vi "NI-Digital Burst Pattern.vi"() -> ()   [LabVIEW 2021]
doc: "Overview\nDemonstrates bursting a pattern that uses the scan opcode and calling the History RAM Fetch Scan Cycle Numbers API."
uses:
  <instrlib>/niDigital/niDigital.llb/niDigital Selected Function.ctl
  <vilib>/Utility/file.llb/Write Delimited Spreadsheet (string).vi
  <instrlib>/niDigital/niDigital.llb/niDigital Fetch History RAM Cycle Information (1D Pin States).vi
  <instrlib>/niDigital/niDigital.llb/niDigital Configure First Failure History RAM Trigger.vi
  <instrlib>/niDigital/niDigital.llb/niDigital Load Specifications Levels and Timing (Single).vi
  <instrlib>/niDigital/niDigital.llb/niDigital Get Pattern Pin List.vi
  <instrlib>/niDigital/niDigital.llb/niDigital Get Pattern Pin Names.vi
  <instrlib>/niDigital/niDigital.llb/niDigital Burst Pattern (Pass Fail).vi
  <instrlib>/niDigital/niDigital.llb/niDigital Pin State.ctl
  <instrlib>/niDigital/niDigital.llb/niDigital History RAM Cycle Information (1D Pin States).ctl
panel:
  in  "Simulate?":bool=TRUE
  in  "resource name":refnum<k15>="PXI1Slot2,PXI1Slot3"
  in  "pretrigger samples":i32
  in  "cycles to acquire":u16(ring)=2303 items=["Failed Cycles"=2303, "All Cycles"=2304]
  out "History RAM cycle information":T1[](array[typedef]) {"actual pin states" items=["0"=0, "1"=1, "L"=3, "H"=4, "X"=5, "M"=6, "V"=7, "D"=8]; "expected pin states" items=["0"=0, "1"=1, "L"=3, "H"=4, "X"=5, "M"=6, "V"=7, "D"=8]}
  out "history RAM sample count":i64
  # "Overview\nDemonstrates bursting a pattern that uses the scan opcode and calling the History RAM Fetch Scan Cycle Numbers API.\n\nInstructions\n1. Use the resource name control to select the digital pattern instrument. Ensure that the instrument name in the PinMap.pinmap file matches the resource name of the digital pattern instrument. The default value for the resource name is \"PXI1Slot2,PXI1Slot3\".\n2. Use the cycles to acquire control to select whether to acquire \"Failed Cycles\" or \"All Cycles\". \n3. Specify the number of pretrigger samples for the History RAM acquisition. \n4. Run the VI.\n5. To run on hardware deselect Simulate? and modify the resource name as appropriate."
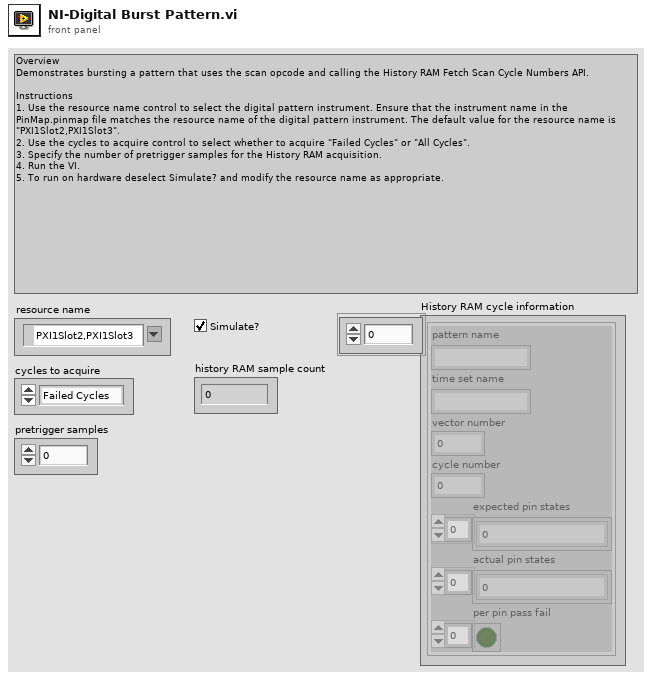
[diagram p1: front panel]
types:
  T1 = typedef "niDigital History RAM Cycle Information (1D Pin States).ctl" = cluster{"pattern name":string, "time set name":string, "vector number":i64, "cycle number":i64, "expected pin states":T2[], "actual pin states":T2[], "per pin pass fail":bool[]}
  T2 = typedef "niDigital Pin State.ctl" = u8
  T3 = typedef "niDigital Selected Function.ctl" = i32
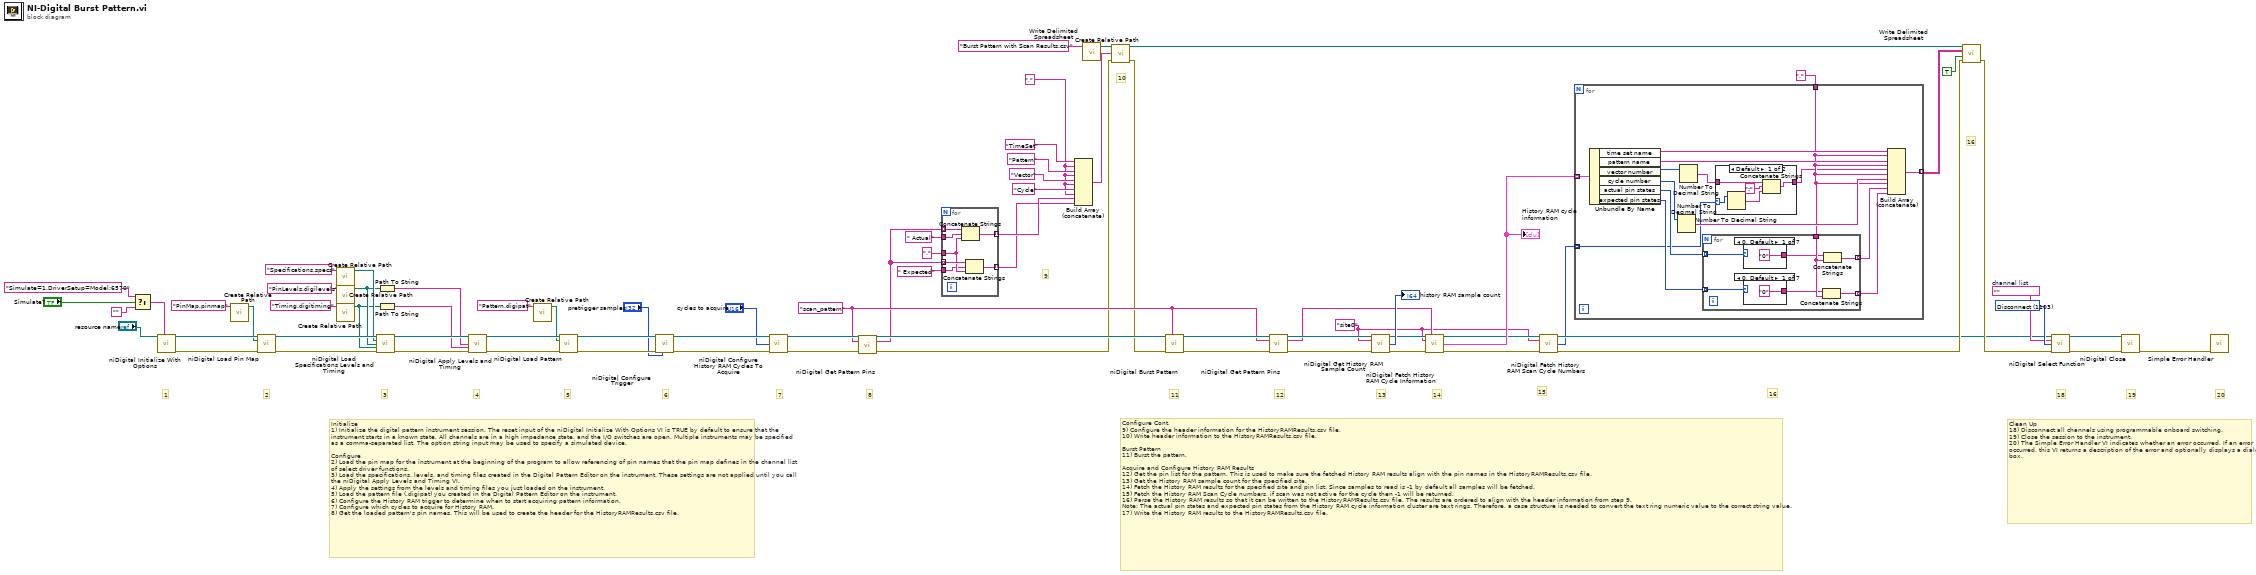
[diagram p0: block diagram]
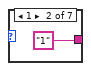
[diagram p3: hidden frame]
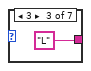
[diagram p4: hidden frame]
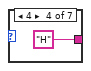
[diagram p5: hidden frame]
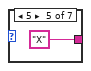
[diagram p6: hidden frame]
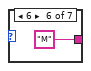
[diagram p7: hidden frame]
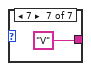
[diagram p8: hidden frame]
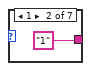
[diagram p9: hidden frame]
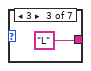
[diagram p10: hidden frame]
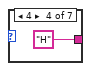
[diagram p11: hidden frame]
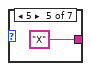
[diagram p12: hidden frame]
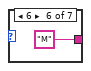
[diagram p13: hidden frame]
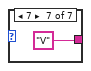
[diagram p14: hidden frame]
diagram:
  w1 = "site0" ("site")
  w28 = "," ("string")
  w40 = "scan_pattern" ("start label")
  w63 = ""  # channel list
  w66 = T3 1103 items=["Digital"=1100, "PPMU"=1101, "Off"=1102, "Disconnect"=1103] ("function")
  # "16"
  # "20"
  # "19"
  # "18"
  # "16"
  # "15"
  # "14"
  # "13"
  # "12"
  # "11"
  # "10"
  # "9"
  # "8"
  # "7"
  # "6"
  # "Clean Up\n18) Disconnect all channels using programmable onboard switching. \n19) Close the session to the instrument.\n20) The Simple Error Handler VI indicates whether an error occurred. If an error occurred, this VI returns a description of the error and optionally displays a dialog box."
  # "Configure Cont.\n9) Configure the header information for the HistoryRAMResults.csv file.\n10) Write header information to the HistoryRAMResults.csv file.\n\nBurst Pattern\n11) Burst the pattern.\n\nAcquire and Configure History RAM Results\n12) Get the pin list for the pattern. This is used to make sure the fetched History RAM results align with the pin names in the HistoryRAMResults.csv file.\n13) Get the History RAM sample count for the specified site.\n14) Fetch the History RAM results for the specified site and pin list. Since samples to read is -1 by default all samples will be fetched.\n15) Fetch the History RAM Scan Cycle numbers, if scan was not active for the cycle then -1 will be returned.\n16) Parse the History RAM results so that it can be written to the HistoryRAMResults.csv file. The results are ordered to align with the header information from step 9. \nNote: The actual pin states and expected pin states from the History RAM cycle information cluster are text rings. Therefore, a case structure is needed to convert the text ring numeric value to the correct string value.\n17) Write the History RAM results to the HistoryRAMResults.csv file."
  # "Initialize\n1) Initialize the digital pattern instrument session. The reset input of the niDigital Initialize With Options VI is TRUE by default to ensure that the instrument starts in a known state. All channels are in a high impedance state, and the I/O switches are open. Multiple instruments may be specified as a comma-separated list. The option string input may be used to specify a simulated device.\n\nConfigure\n2) Load the pin map for the instrument at the beginning of the program to allow referencing of pin names that the pin map defines in the channel list of select driver functions.\n3) Load the specifications, levels, and timing files created in the Digital Pattern Editor on the instrument. These settings are not applied until you call the niDigital Apply Levels and Timing VI.\n4) Apply the settings from the levels and timing files you just loaded on the instrument.\n5) Load the pattern file (.digipat) you created in the Digital Pattern Editor on the instrument.\n6) Configure the History RAM trigger to determine when to start acquiring pattern information.\n7) Configure which cycles to acquire for History RAM.\n8) Get the loaded pattern's pin names. This will be used to create the header for the HistoryRAMResults.csv file."
  # "5"
  # "4"
  # "3"
  # "2"
  # "1"
  n1 = Select(t="Simulate=1,DriverSetup=Model:6570", s="Simulate?", f="") -> (s? t:f=w7:string)
  n2 = call <instrlib>:"niDigital Initialize With Options.vi"("resource name"="resource name", "option string"=w7) -> ("instrument handle"=w71:refnum<k15>, "error out"=w70:errorcluster)  [unwired: 12 in]
  n3 = call "Create Relative Path.vi"("file name"="PinMap.pinmap" ("name or relative path")) -> ("appended path"=w61:path)  [unwired: 4 in]
  n4 = call <instrlib>:"niDigital Load Pin Map.vi"("instrument handle"=w71, "pin map file"=w61, "error in"=w70) -> ("instrument handle out"=w68:refnum<k15>, "error out"=w67:errorcluster)  [unwired: 11 in]
  n5 = call "Create Relative Path.vi"("file name"="Specifications.specs" ("name or relative path")) -> ("appended path"=w58:path)  [unwired: 4 in]
  n6 = call "Create Relative Path.vi"("file name"="PinLevels.digilevels" ("name or relative path")) -> ("appended path"=w57:path)  [unwired: 4 in]
  n7 = call "Create Relative Path.vi"("file name"="Timing.digitiming" ("name or relative path")) -> ("appended path"=w56:path)  [unwired: 4 in]
  n8 = call-poly <instrlib>:"niDigital Load Specifications Levels and Timing.vi"("instrument handle"=w68, "specifications file path"=w58, "levels file path"=w57, "timing file path"=w56, "error in"=w67) -> ("instrument handle out"=w76:refnum<k15>, "error out"=w75:errorcluster)  [unwired: 9 in]
  n9 = Path To String(path=w57) -> (string=w69:string)
  n10 = Path To String(path=w56) -> (string=w72:string)
  n11 = call <instrlib>:"niDigital Apply Levels and Timing.vi"("instrument handle"=w76, "levels sheet"=w69, "timing sheet"=w72, "error in"=w75) -> ("instrument handle out"=w73:refnum<k15>, "error out"=w74:errorcluster)  [unwired: 10 in]
  n12 = call "Create Relative Path.vi"("file name"="Pattern.digipat" ("name or relative path")) -> ("appended path"=w54:path)  [unwired: 4 in]
  n13 = call <instrlib>:"niDigital Load Pattern.vi"("instrument handle"=w73, "pattern file"=w54, "error in"=w74) -> ("instrument handle out"=w52:refnum<k15>, "error out"=w51:errorcluster)  [unwired: 11 in]
  n14 = call-poly <instrlib>:"niDigital Configure Trigger.vi"("instrument handle"=w52, "error in"=w51, "pretrigger samples"="pretrigger samples") -> ("instrument handle out"=w49:refnum<k15>, "error out"=w50:errorcluster)  [unwired: 11 in]
  n15 = call <instrlib>:"niDigital Configure History RAM Cycles To Acquire.vi"("instrument handle"=w49, "cycles to acquire"="cycles to acquire", "error in"=w50) -> ("instrument handle out"=w43:refnum<k15>, "error out"=w42:errorcluster)  [unwired: 11 in]
  n16 = call-poly <instrlib>:"niDigital Get Pattern Pins.vi"("instrument handle"=w43, "start label"=w40, "error in"=w42) -> ("instrument handle out"=w41:refnum<k15>, "pin names"=w39:string[], "error out"=w17:errorcluster)  [unwired: 10 in]
  n17 = for {
    tunnel: w39 -> [w83] mode=indexing
    tunnel: [w82] -> w38 mode=indexing
    tunnel: w39 -> [w80] mode=indexing
    tunnel: [w81] -> w37 mode=indexing
    tunnel: " Actual" ("string") -> [w79]
    tunnel: "," ("string") -> [w78]
    tunnel: " Expected" ("string") -> [w77]
    n18 = Concatenate Strings(w83, w79, w78) -> (w82:string)
    n19 = Concatenate Strings(w80, w77, w78) -> (w81:string)
  }
  n20 = Build Array (concatenate)("TimeSet", w28, "Pattern" ("element"), w28, "Vector" ("element"), w28, "Cycle" ("element"), w28, w38, w37) -> (w36:string[])
  n21 = call "Create Relative Path.vi"("file name"="Burst Pattern with Scan Results.csv") -> ("appended path"=w30:path)  [unwired: 4 in]
  n22 = call-poly <vilib>:"Write Delimited Spreadsheet.vi"("file path (dialog if empty)"=w30, "1D data"=w36, "error in (no error)"=w17) -> ("new file path (Not A Path if cancelled)"=w29:path, "error out"=w16:errorcluster)  [unwired: 11 in]
  n23 = call-poly <instrlib>:"niDigital Burst Pattern.vi"("instrument handle"=w41, "start label"=w40, "error in"=w16) -> ("instrument handle out"=w46:refnum<k15>, "error out"=w47:errorcluster)  [unwired: 10 in, 1 out]
  n24 = call-poly <instrlib>:"niDigital Get Pattern Pins.vi"("instrument handle"=w46, "start label"=w40, "error in"=w47) -> ("instrument handle out"=w45:refnum<k15>, "pin list"=w22:string, "error out"=w44:errorcluster)  [unwired: 10 in]
  n25 = call <instrlib>:"niDigital Get History RAM Sample Count.vi"("instrument handle"=w45, "site"=w1, "error in"=w44) -> ("instrument handle out"=w6:refnum<k15>, "sample count"=→"history RAM sample count":i64, "error out"=w48:errorcluster)  [unwired: 10 in]
  n26 = call-poly <instrlib>:"niDigital Fetch History RAM Cycle Information.vi"("instrument handle"=w6, "pin list"=w22, "site"=w1, "error in"=w48) -> ("instrument handle out"=w4:refnum<k15>, "cycle information"=w24:T1[], "error out"=w15:errorcluster)  [unwired: 9 in]
  "History RAM cycle information" <- w24
  n27 = call <instrlib>:"niDigital Fetch History RAM Scan Cycle Numbers.vi"("instrument handle"=w4, "site"=w1, "error in"=w15) -> ("instrument handle out"=w3:refnum<k15>, "scan cycle numbers"=w2:i64[], "error out"=w5:errorcluster)  [unwired: 10 in]
  n28 = for {
    tunnel: w24 -> [w98] mode=indexing
    tunnel: [w92] -> w27 mode=indexing
    tunnel: "," ("element") -> [w89]
    tunnel: w2 -> [w84] mode=indexing
    n29 = Unbundle By Name(w98) -> ("time set name"=w97:string, "pattern name"=w96:string, "vector number"=w87:i64, "cycle number"=w88:i64, "actual pin states"=w90:T2[], "expected pin states"=w91:T2[])
    n30 = Number To Decimal String(number=w88) -> (decimal integer string=w95:string)  [unwired: 1 in]
    n31 = Number To Decimal String(number=w87) -> (decimal integer string=w86:string)  [unwired: 1 in]
    n32 = for {
      tunnel: w91 -> [w107] mode=indexing
      tunnel: [w111] -> w94 mode=indexing
      tunnel: [w110] -> w93 mode=indexing
      tunnel: w90 -> [w108] mode=indexing
      tunnel: w89 -> [w109]
      n33 = case shown="0, Default" w108 {
        tunnel: ["0" ("element") "1" ("element") "L" ("element") "H" ("element") "X" ("element") "M" ("element") "V" ("element")] -> w106
        frame 0, Default {
        }
        frame 1 {
        }
        frame 3 {
        }
        frame 4 {
        }
        frame 5 {
        }
        frame 6 {
        }
        frame 7 {
        }
      }
      n34 = case shown="0, Default" w107 {
        tunnel: ["0" ("element") "1" ("element") "L" ("element") "H" ("element") "X" ("element") "M" ("element") "V" ("element")] -> w105
        frame 0, Default {
        }
        frame 1 {
        }
        frame 3 {
        }
        frame 4 {
        }
        frame 5 {
        }
        frame 6 {
        }
        frame 7 {
        }
      }
      n35 = Concatenate Strings(w105, w109) -> (w110:string)
      n36 = Concatenate Strings(w106, w109) -> (w111:string)
    }
    n37 = case shown="Default" w84 {
      selector: w84 -> [w99 _]
      tunnel: w86 -> [w102 w104]
      tunnel: [w103 w104] -> w85
      frame Default {
        n38 = Number To Decimal String(number=w99) -> (decimal integer string=w100:string)  [unwired: 1 in]
        n39 = Concatenate Strings(w102, ":" ("string"), w100) -> (w103:string)
      }
      frame -1 {
      }
    }
    n40 = Build Array (concatenate)(w97, w89, w96, w89, w85, w89, w95, w89, w94, w93) -> (w92:string[])
  }
  n41 = call-poly <vilib>:"Write Delimited Spreadsheet.vi"("file path (dialog if empty)"=w29, "2D data"=w27, "append to file? (new file:F)"=TRUE ("append to file? (F)"), "error in (no error)"=w5) -> ("error out"=w14:errorcluster)  [unwired: 10 in, 1 out]
  n42 = call <instrlib>:"niDigital Select Function.vi"("instrument handle"=w3, "channel list"=w63, "function"=w66, "error in"=w14) -> ("instrument handle out"=w65:refnum<k15>, "error out"=w64:errorcluster)  [unwired: 10 in]
  n43 = call <instrlib>:"niDigital Close.vi"("instrument handle"=w65, "error in"=w64) -> ("error out"=w13:errorcluster)  [unwired: 13 in]
  n44 = call <vilib>:"Simple Error Handler.vi"("error in (no error)"=w13) -> ()  [unwired: 4 in, 5 out]
